vi "Write Step Analyze.vi"(11 "AC Advance Step Data":T1 {"Transient Time" format="%.1f ms"; "Transient Site" format="%.0f ¢X"; "Transient Volt" format="%.1f V"; "CF Lo Limit" format="%.2f"; "CF Hi Limit" format="%.2f"; "Q Lo Limit" format="%.0f VAR"; "Q Hi Limit" format="%.0f VAR"; "VA Lo Limit" format="%.0f VA"; "VA Hi Limit" format="%.0f VA"; "PF Lo Limit" format="%.3f"; "PF Hi Limit" format="%.3f"; "P Lo Limit" format="%.0f W"; "P Hi Limit" format="%.0f W"; "AP Lo Limit" format="%.1f A"; "AP Hi Limit" format="%.1f A"; "A Lo Limit" format="%.2f A"; "A Hi Limit" format="%.2f A"; "Delay Time" format="%.1f s"; "£GT" format="%.0f ms"; "£GF" format="%.1f Hz"; "£GV" format="%.1f V"; "Time" format="%.1f s"; "Voltage" format="%.1f V"; "Frequency" format="%.1f Hz"}) -> (3 "Data":string)   [LabVIEW 2013]
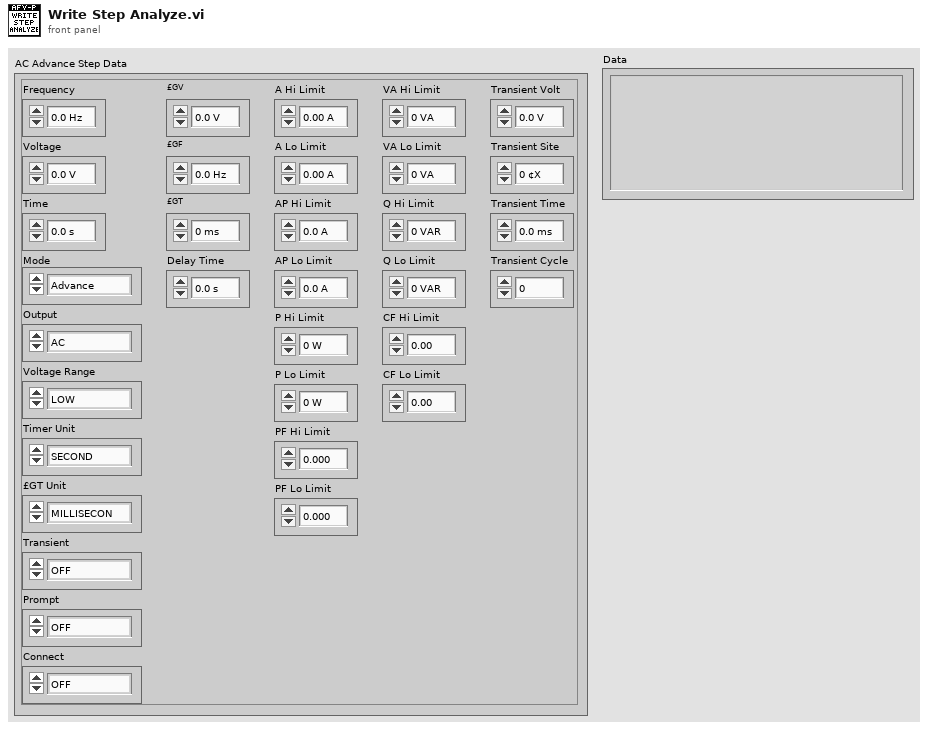
[diagram p1: front panel]
types:
  T1 = cluster{"Frequency":dbl, "Voltage":dbl, "Time":dbl, "Mode":enum16{"Advance", "Basic"}, "Output":enum16{"AC", "DC"}, "Voltage Range":enum16{"LOW", "HIGH", "AUTO"}, "Timer Unit":enum16{"SECOND", "MINUTE", "HOUR"}, "£GT Unit":enum16{"MILLISECON", "SECOND", "CYCLE"}, "Transient":enum16{"OFF", "ON"}, "Prompt":enum16{"OFF", "ON"}, "Connect":enum16{"OFF", "ON"}, "£GV":dbl, "£GF":dbl, "£GT":u16, "Delay Time":dbl, "A Hi Limit":dbl, "A Lo Limit":dbl, "AP Hi Limit":dbl, "AP Lo Limit":dbl, "P Hi Limit":u16, "P Lo Limit":u16, "PF Hi Limit":dbl, "PF Lo Limit":dbl, "VA Hi Limit":u16, "VA Lo Limit":u16, "Q Hi Limit":u16, "Q Lo Limit":u16, "CF Hi Limit":dbl, "CF Lo Limit":dbl, "Transient Volt":dbl, "Transient Site":u16, "Transient Time":dbl, "Transient Cycle":u16}
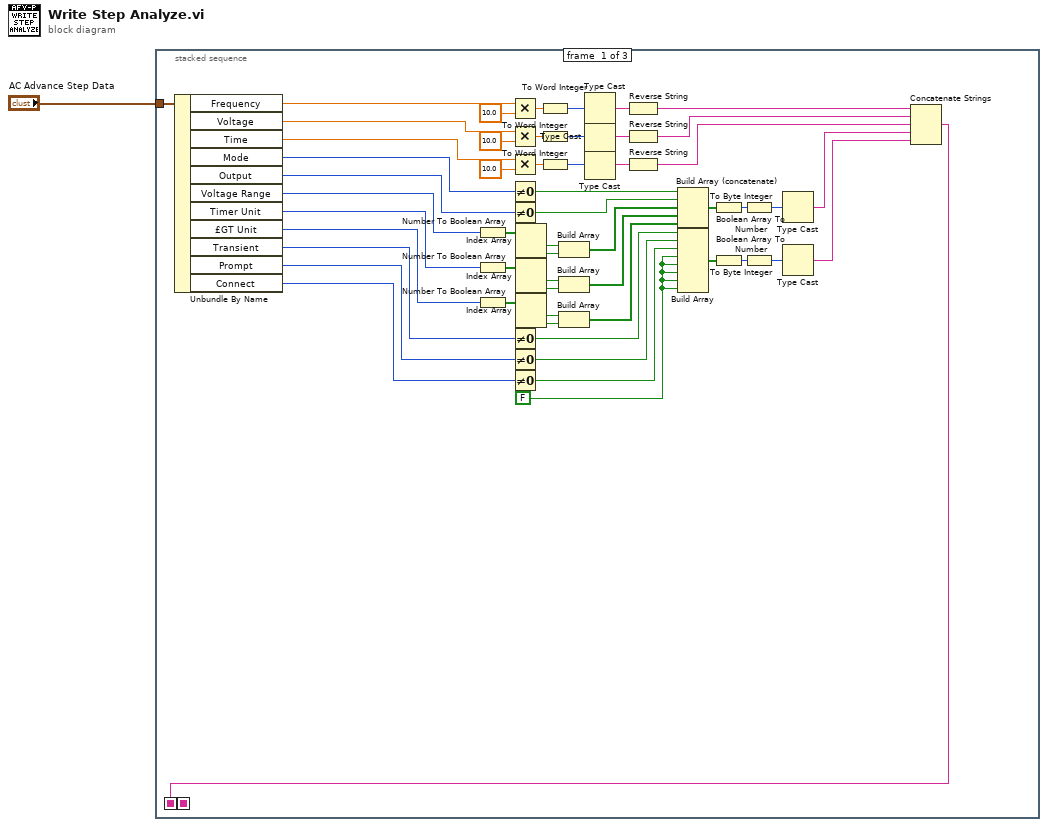
[diagram p0: block diagram]
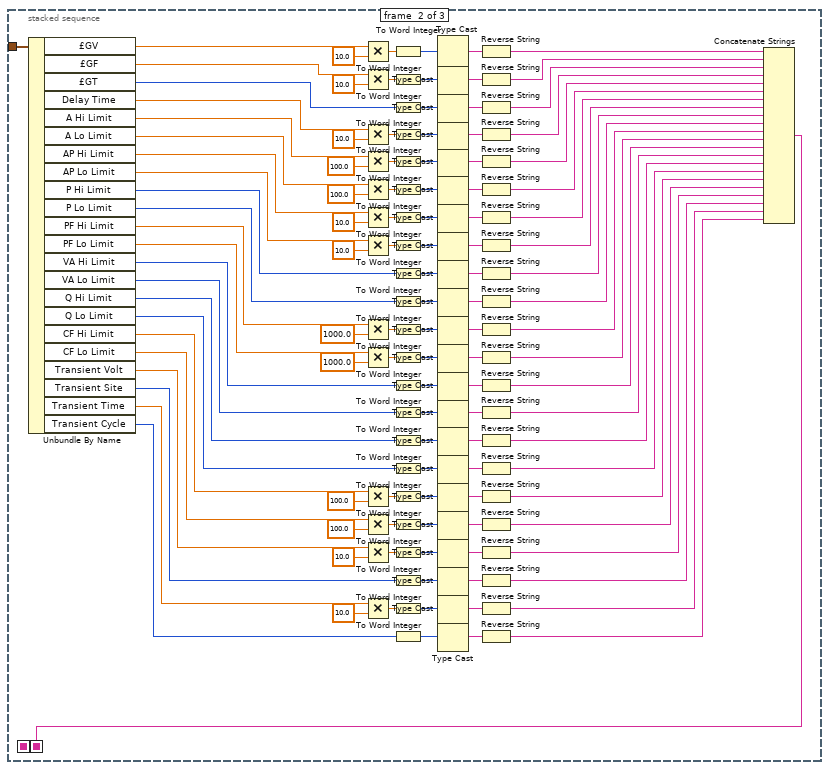
[diagram p2: hidden frame]
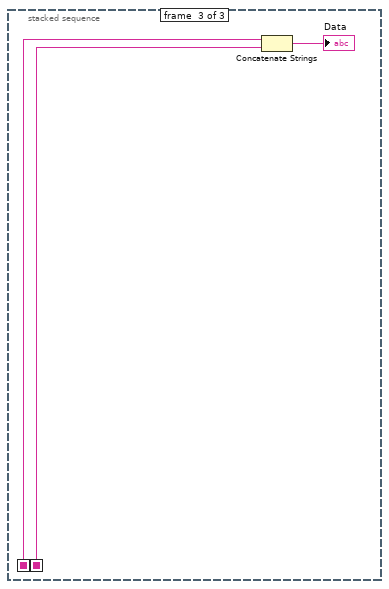
[diagram p3: hidden frame]
diagram:
  n1 = stacked-sequence {
    seq-local: [w4 _ _] -> [_ _ w174]
    seq-local: [_ w155 _] -> [_ _ w173]
    tunnel: "AC Advance Step Data" -> [w55 w171 _]
    frame #0 {
      w10 = FALSE ("element")
      n2 = Unbundle By Name(w55) -> ("Frequency"=w54:dbl, "Voltage"=w45:dbl, "Time"=w40:dbl, "Mode"=w32:enum16{"Advance", "Basic"}, "Output"=w39:enum16{"AC", "DC"}, "Voltage Range"=w25:enum16{"LOW", "HIGH", "AUTO"}, "Timer Unit"=w20:enum16{"SECOND", "MINUTE", "HOUR"}, "£GT Unit"=w15:enum16{"MILLISECON", "SECOND", "CYCLE"}, "Transient"=w38:enum16{"OFF", "ON"}, "Prompt"=w37:enum16{"OFF", "ON"}, "Connect"=w36:enum16{"OFF", "ON"})
      n3 = Number To Boolean Array(number=w25) -> (Boolean array=w31:bool[])
      n4 = Number To Boolean Array(number=w20) -> (Boolean array=w21:bool[])
      n5 = Number To Boolean Array(number=w15) -> (Boolean array=w18:bool[])
      n6 = Multiply(x=w54, y=10.0) -> (x*y=w52:dbl)
      n7 = Multiply(x=w45, y=10.0) -> (x*y=w47:dbl)
      n8 = Multiply(x=w40, y=10.0) -> (x*y=w43:dbl)
      n9 = Not Equal To 0?(x=w32) -> (x != 0?=w35:bool)
      n10 = Not Equal To 0?(x=w39) -> (x != 0?=w34:bool)
      n11 = Not Equal To 0?(x=w38) -> (x != 0?=w13:bool)
      n12 = Not Equal To 0?(x=w37) -> (x != 0?=w12:bool)
      n13 = Not Equal To 0?(x=w36) -> (x != 0?=w11:bool)
      n14 = Index Array(array=w31) -> (element #1=w30:bool, element #2=w29:bool)  [unwired: 2 in]
      n15 = Index Array(array=w21) -> (element #1=w22:bool, element #2=w23:bool)  [unwired: 2 in]
      n16 = Index Array(array=w18) -> (element #1=w17:bool, element #2=w16:bool)  [unwired: 2 in]
      n17 = To Word Integer(number=w52) -> (16bit integer=w51:i16)
      n18 = To Word Integer(number=w47) -> (16bit integer=w48:i16)
      n19 = To Word Integer(number=w43) -> (16bit integer=w42:i16)
      n20 = Build Array(w30, w29) -> (w24:bool[])
      n21 = Build Array(w22, w23) -> (w19:bool[])
      n22 = Build Array(w17, w16) -> (w14:bool[])
      n23 = Type Cast(x=w51) -> (*(type *) &x=w50:string)  [unwired: 1 in]
      n24 = Type Cast(x=w48) -> (*(type *) &x=w49:string)  [unwired: 1 in]
      n25 = Type Cast(x=w42) -> (*(type *) &x=w41:string)  [unwired: 1 in]
      n26 = Reverse String(1:w50) -> (0:w28:string)
      n27 = Reverse String(1:w49) -> (0:w27:string)
      n28 = Reverse String(1:w41) -> (0:w26:string)
      n29 = Build Array (concatenate)(w35, w34, w24, w19, w14) -> (w33:bool[])
      n30 = Build Array(w13, w12, w11, w10, w10, w10, w10, w10) -> (w9:bool[])
      n31 = Boolean Array To Number(Boolean array=w33) -> (number=w8:u32)
      n32 = Boolean Array To Number(Boolean array=w9) -> (number=w5:u32)
      n33 = To Byte Integer(number=w8) -> (8bit integer=w7:i8)
      n34 = To Byte Integer(number=w5) -> (8bit integer=w6:i8)
      n35 = Type Cast(x=w7) -> (*(type *) &x=w3:string)  [unwired: 1 in]
      n36 = Type Cast(x=w6) -> (*(type *) &x=w2:string)  [unwired: 1 in]
      n37 = Concatenate Strings(w28, w27, w26, w3, w2) -> (w4:string)
    }
    frame #1 {
      n38 = Unbundle By Name(w171) -> ("£GV"=w170:dbl, "£GF"=w161:dbl, "£GT"=w154:u16, "Delay Time"=w149:dbl, "A Hi Limit"=w142:dbl, "A Lo Limit"=w136:dbl, "AP Hi Limit"=w125:dbl, "AP Lo Limit"=w124:dbl, "P Hi Limit"=w117:u16, "P Lo Limit"=w116:u16, "PF Hi Limit"=w107:dbl, "PF Lo Limit"=w106:dbl, "VA Hi Limit"=w95:u16, "VA Lo Limit"=w94:u16, "Q Hi Limit"=w93:u16, "Q Lo Limit"=w92:u16, "CF Hi Limit"=w79:dbl, "CF Lo Limit"=w78:dbl, "Transient Volt"=w71:dbl, "Transient Site"=w67:u16, "Transient Time"=w61:dbl, "Transient Cycle"=w57:u16)
      n39 = Multiply(x=w170, y=10.0) -> (x*y=w168:dbl)
      n40 = Multiply(x=w161, y=10.0) -> (x*y=w163:dbl)
      n41 = Multiply(x=w149, y=10.0) -> (x*y=w151:dbl)
      n42 = Multiply(x=w142, y=100.0) -> (x*y=w146:dbl)
      n43 = Multiply(x=w136, y=100.0) -> (x*y=w139:dbl)
      n44 = Multiply(x=w125, y=10.0) -> (x*y=w129:dbl)
      n45 = Multiply(x=w124, y=10.0) -> (x*y=w134:dbl)
      n46 = Multiply(x=w107, y=1000.0) -> (x*y=w114:dbl)
      n47 = Multiply(x=w106, y=1000.0) -> (x*y=w109:dbl)
      n48 = Multiply(x=w79, y=100.0) -> (x*y=w81:dbl)
      n49 = Multiply(x=w78, y=100.0) -> (x*y=w86:dbl)
      n50 = Multiply(x=w71, y=10.0) -> (x*y=w73:dbl)
      n51 = Multiply(x=w61, y=10.0) -> (x*y=w64:dbl)
      n52 = To Word Integer(number=w168) -> (16bit integer=w167:i16)
      n53 = To Word Integer(number=w163) -> (16bit integer=w164:i16)
      n54 = To Word Integer(number=w154) -> (16bit integer=w160:i16)
      n55 = To Word Integer(number=w151) -> (16bit integer=w152:i16)
      n56 = To Word Integer(number=w146) -> (16bit integer=w145:i16)
      n57 = To Word Integer(number=w139) -> (16bit integer=w140:i16)
      n58 = To Word Integer(number=w129) -> (16bit integer=w130:i16)
      n59 = To Word Integer(number=w134) -> (16bit integer=w133:i16)
      n60 = To Word Integer(number=w117) -> (16bit integer=w122:i16)
      n61 = To Word Integer(number=w116) -> (16bit integer=w121:i16)
      n62 = To Word Integer(number=w114) -> (16bit integer=w113:i16)
      n63 = To Word Integer(number=w109) -> (16bit integer=w110:i16)
      n64 = To Word Integer(number=w95) -> (16bit integer=w101:i16)
      n65 = To Word Integer(number=w94) -> (16bit integer=w102:i16)
      n66 = To Word Integer(number=w93) -> (16bit integer=w98:i16)
      n67 = To Word Integer(number=w92) -> (16bit integer=w97:i16)
      n68 = To Word Integer(number=w81) -> (16bit integer=w82:i16)
      n69 = To Word Integer(number=w86) -> (16bit integer=w85:i16)
      n70 = To Word Integer(number=w73) -> (16bit integer=w74:i16)
      n71 = To Word Integer(number=w67) -> (16bit integer=w68:i16)
      n72 = To Word Integer(number=w64) -> (16bit integer=w63:i16)
      n73 = To Word Integer(number=w57) -> (16bit integer=w59:i16)
      n74 = Type Cast(x=w167) -> (*(type *) &x=w166:string)  [unwired: 1 in]
      n75 = Type Cast(x=w164) -> (*(type *) &x=w165:string)  [unwired: 1 in]
      n76 = Type Cast(x=w160) -> (*(type *) &x=w159:string)  [unwired: 1 in]
      n77 = Type Cast(x=w152) -> (*(type *) &x=w153:string)  [unwired: 1 in]
      n78 = Type Cast(x=w145) -> (*(type *) &x=w144:string)  [unwired: 1 in]
      n79 = Type Cast(x=w140) -> (*(type *) &x=w141:string)  [unwired: 1 in]
      n80 = Type Cast(x=w130) -> (*(type *) &x=w131:string)  [unwired: 1 in]
      n81 = Type Cast(x=w133) -> (*(type *) &x=w132:string)  [unwired: 1 in]
      n82 = Type Cast(x=w122) -> (*(type *) &x=w123:string)  [unwired: 1 in]
      n83 = Type Cast(x=w121) -> (*(type *) &x=w120:string)  [unwired: 1 in]
      n84 = Type Cast(x=w113) -> (*(type *) &x=w112:string)  [unwired: 1 in]
      n85 = Type Cast(x=w110) -> (*(type *) &x=w111:string)  [unwired: 1 in]
      n86 = Type Cast(x=w101) -> (*(type *) &x=w100:string)  [unwired: 1 in]
      n87 = Type Cast(x=w102) -> (*(type *) &x=w103:string)  [unwired: 1 in]
      n88 = Type Cast(x=w98) -> (*(type *) &x=w99:string)  [unwired: 1 in]
      n89 = Type Cast(x=w97) -> (*(type *) &x=w96:string)  [unwired: 1 in]
      n90 = Type Cast(x=w82) -> (*(type *) &x=w83:string)  [unwired: 1 in]
      n91 = Type Cast(x=w85) -> (*(type *) &x=w84:string)  [unwired: 1 in]
      n92 = Type Cast(x=w74) -> (*(type *) &x=w75:string)  [unwired: 1 in]
      n93 = Type Cast(x=w68) -> (*(type *) &x=w69:string)  [unwired: 1 in]
      n94 = Type Cast(x=w63) -> (*(type *) &x=w62:string)  [unwired: 1 in]
      n95 = Type Cast(x=w59) -> (*(type *) &x=w58:string)  [unwired: 1 in]
      n96 = Reverse String(1:w166) -> (0:w158:string)
      n97 = Reverse String(1:w165) -> (0:w157:string)
      n98 = Reverse String(1:w159) -> (0:w156:string)
      n99 = Reverse String(1:w153) -> (0:w148:string)
      n100 = Reverse String(1:w144) -> (0:w143:string)
      n101 = Reverse String(1:w141) -> (0:w137:string)
      n102 = Reverse String(1:w131) -> (0:w127:string)
      n103 = Reverse String(1:w132) -> (0:w126:string)
      n104 = Reverse String(1:w123) -> (0:w119:string)
      n105 = Reverse String(1:w120) -> (0:w118:string)
      n106 = Reverse String(1:w112) -> (0:w105:string)
      n107 = Reverse String(1:w111) -> (0:w104:string)
      n108 = Reverse String(1:w100) -> (0:w91:string)
      n109 = Reverse String(1:w103) -> (0:w90:string)
      n110 = Reverse String(1:w99) -> (0:w89:string)
      n111 = Reverse String(1:w96) -> (0:w88:string)
      n112 = Reverse String(1:w83) -> (0:w77:string)
      n113 = Reverse String(1:w84) -> (0:w76:string)
      n114 = Reverse String(1:w75) -> (0:w70:string)
      n115 = Reverse String(1:w69) -> (0:w66:string)
      n116 = Reverse String(1:w62) -> (0:w60:string)
      n117 = Reverse String(1:w58) -> (0:w56:string)
      n118 = Concatenate Strings(w158, w157, w156, w148, w143, w137, w127, w126, w119, w118, w105, w104, w91, w90, w89, w88, w77, w76, w70, w66, w60, w56) -> (w155:string)
    }
    frame #2 {
      n119 = Concatenate Strings(w174, w173) -> (→"Data":string)
    }
  }
